vi "Initialize.vi"(8 "error in":errorcluster, 10 "parameters":variant, 11 "cRIO in":refnum<class "cRIO.lvclass">) -> (0 "error out":errorcluster, 2 "summary":T2[](array[typedef]), 3 "data value reference":T1)   [LabVIEW 2015, in "cRIO.lvclass"]
doc: "This Vi initializes the data of a node its default state.\nThe object is not created inside of this ViI, beacuase it is created from a File depending on user selection."
uses:
  cRIO.lvclass
  <vilib>/NI/Configuration Framework/Node/Summary.ctl
  <vilib>/NI/Configuration Framework/Node/NodeRef.ctl
  <vilib>/NI/Configuration Framework/Node/NISE_CEF_Node.lvclass
  cRIO.lvclass/cRIO.ctl
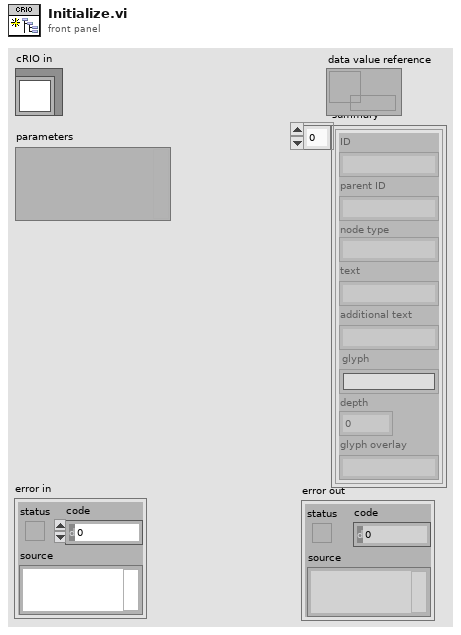
[diagram p1: front panel]
types:
  T1 = typedef "NISE_CEF_Node.lvclass/NodeRef.ctl" = refnum<data-value>
  T2 = typedef "NISE_CEF_Node.lvclass/Summary.ctl" = cluster{"ID":string, "parent ID":string, "node type":string, "text":string, "additional text":string, "glyph":string, "depth":i32, "glyph overlay":string}
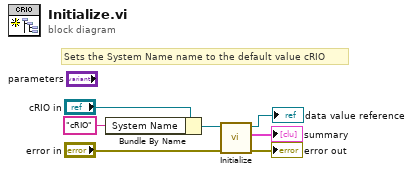
[diagram p0: block diagram]
diagram:
  # "Sets the System Name name to the default value cRIO"
  n1 = Bundle By Name(cluster="cRIO in", "System Name"="cRIO") -> (w3:refnum<class "cRIO.lvclass">)
  n2 = call-parent "Initialize.vi"("error in"="error in", "node in"=w3) -> ("error out"=→"error out":errorcluster, "summary"=→"summary":T2[], "data value reference"=→"data value reference":T1)  [unwired: 7 in]
